vi "Ascensor_parcial1.vi"() -> ()   [LabVIEW 2018]
panel:
  in  "Enum":T1(ring)=enum."Cerrar"
  out "Asc/Desc":i16
  out "Pet Asc":i32[](array[numeric])
  out "Pet Desc":i32[](array[numeric])
  in  "Stop/Start":bool
  in  "Automatico/Manual":bool
  in  "stop":bool
  out "PurtasAux":dbl
  in  "Abierto M":bool
  in  "AbajoM":bool
  in  "Cerrado M":bool
  in  "Sen Puerta":bool
  in  "ArribaM":bool
  out "Elevador":i8(ring) caption="Puertas Elevador"
  in  "Down 2":bool
  in  "Up 2":bool
  in  "Down 3":bool
  in  "Up 3":bool
  in  "Down 4":bool
  in  "Up 1":bool
  in  "Close":bool
  in  "Open":bool
  in  "4":bool
  in  "1":bool
  in  "2":bool
  in  "3":bool
  in  "Display":i8(ring)
  out "Pos S3":i32=477
  out "Pos S4":i32=351
  out "Pos S2":i32=602
  out "Pos S1":i32=730
  in  "S4":bool
  in  "S3":bool
  in  "S2":bool
  in  "S1":bool
  # "Botonera interna"
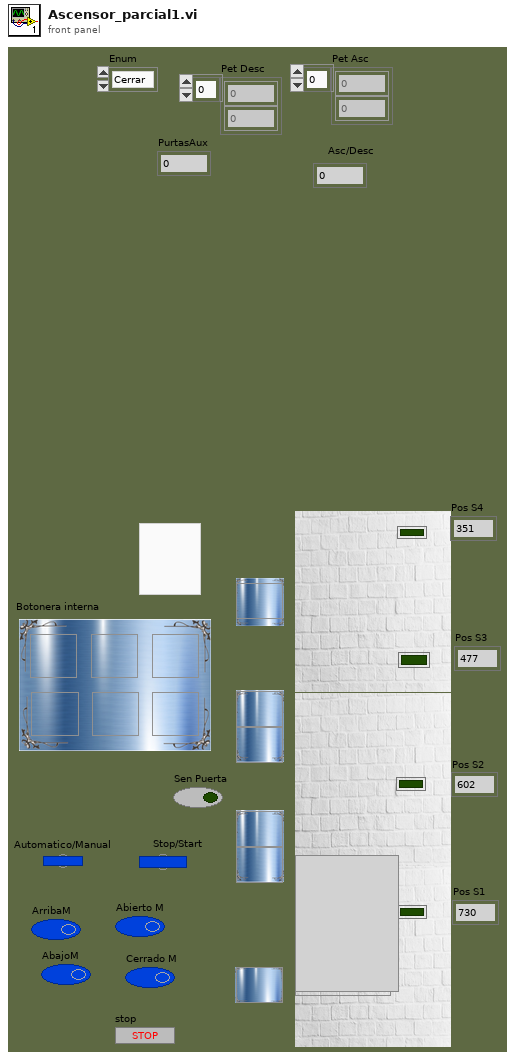
[diagram p1: front panel]
types:
  T1 = enum16{"Abrir", "Cerrar", "Ascender ", "Descender", "Eliminar"}
  T2 = enum16{"Abrir", "Cerrar", "Ascender ", "Descender", ""}
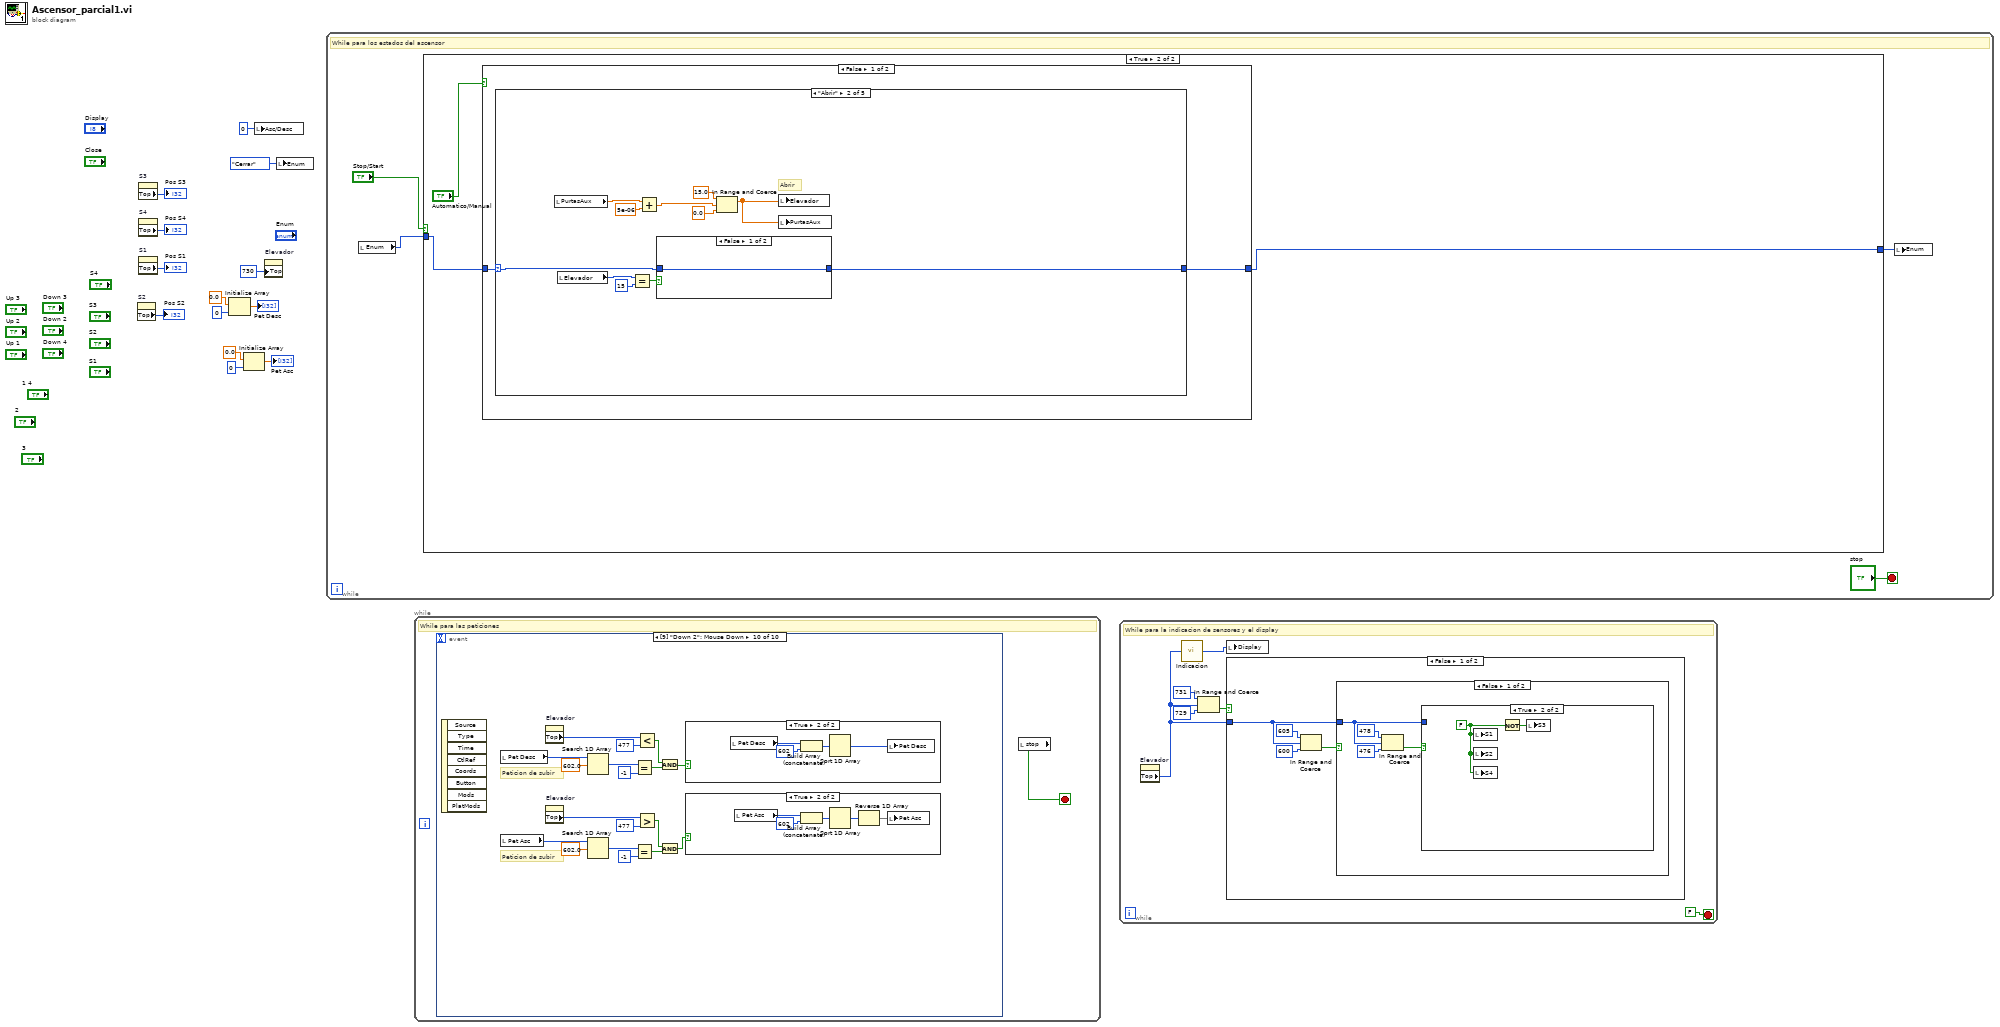
[diagram p0: block diagram]
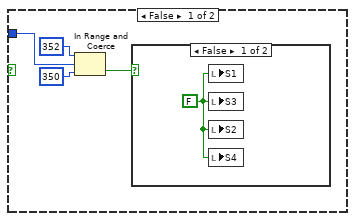
[diagram p2: hidden frame]
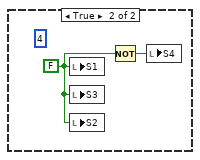
[diagram p3: hidden frame]
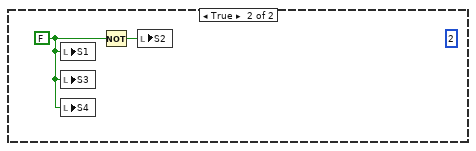
[diagram p4: hidden frame]
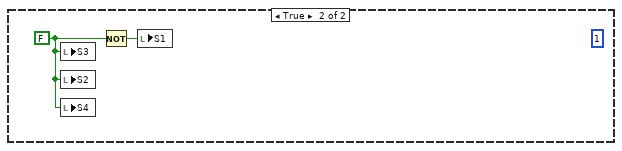
[diagram p5: hidden frame]
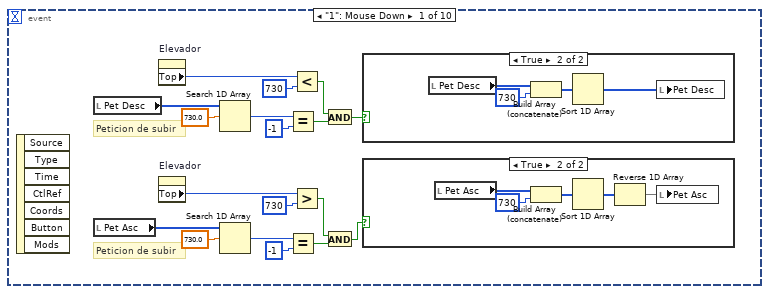
[diagram p6: hidden frame]
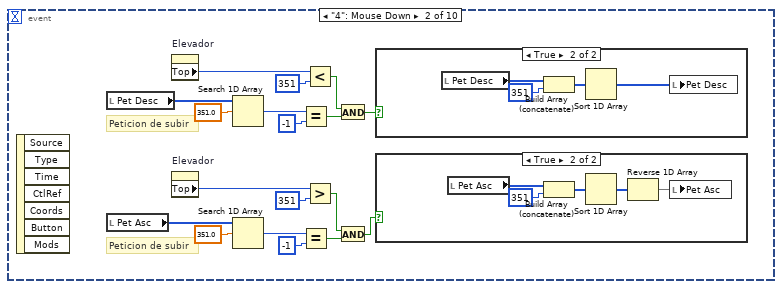
[diagram p9: hidden frame]
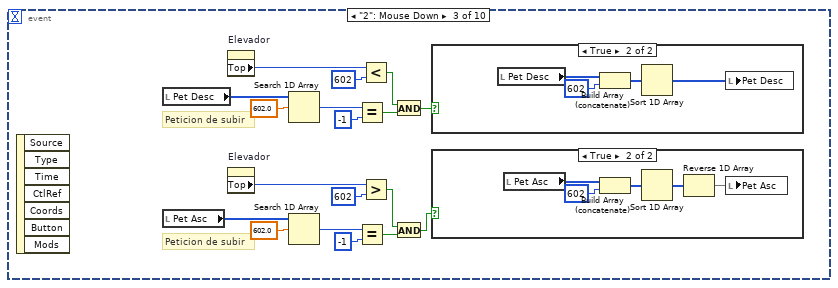
[diagram p12: hidden frame]
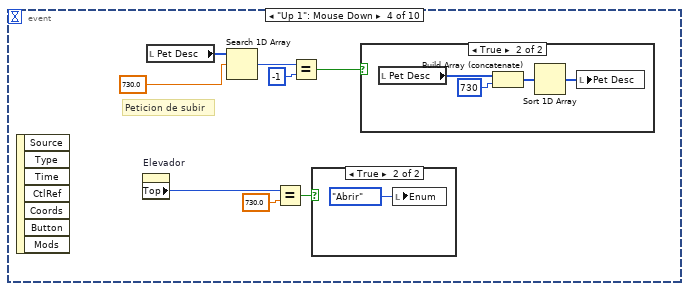
[diagram p15: hidden frame]
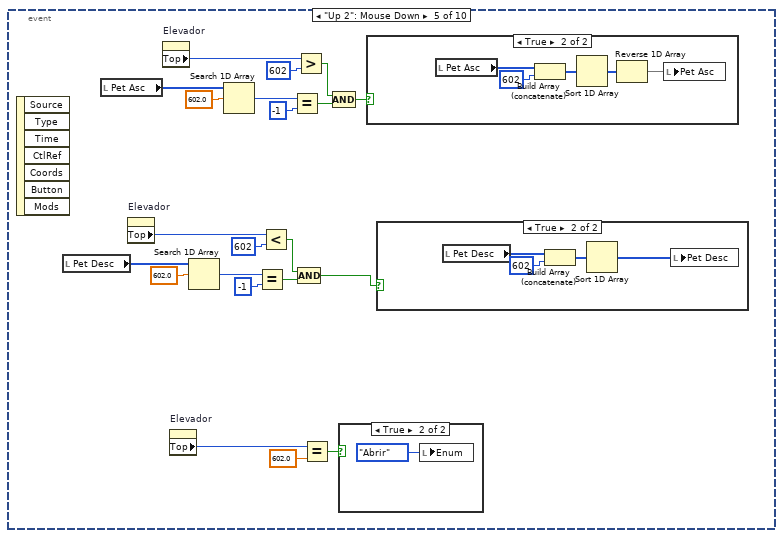
[diagram p18: hidden frame]
diagram:
  n1 = property on="S2" class="Bool (strict)"() -> ("Top"=→"Pos S2":i32)  [unwired: 2 in, 2 out]
  n2 = property on="S3" class="Bool (strict)"() -> ("Top"=→"Pos S3":i32)  [unwired: 2 in, 2 out]
  n3 = property on="S4" class="Bool (strict)"() -> ("Top"=→"Pos S4":i32)  [unwired: 2 in, 2 out]
  n4 = property on="S1" class="Bool (strict)"() -> ("Top"=→"Pos S1":i32)  [unwired: 2 in, 2 out]
  n5 = Initialize Array(0.0 ("element"), 0 ("dimension size")) -> (→"Pet Desc":dbl[])
  n6 = Initialize Array(0.0 ("element"), 0 ("dimension size")) -> (→"Pet Asc":dbl[])
  n7 = local write "Asc/Desc"(i16 0 ("Asc/Desc")) -> ()
  n8 = property on="Elevador" class="Ring (strict)"("Top"=730 ("Position:Top")) -> ()  [unwired: 2 in, 2 out]
  n9 = local write "Enum"(T1."Cerrar" ("Enum")) -> ()
  n10 = while {
    stop <- "stop" stop-if-true
    # "While para los estados del ascensor"
    n11 = local read "Enum"() -> (w15:T1)
    n12 = case shown="True" "Stop/Start" {
      tunnel: w15 -> [_ w20]
      tunnel: [T1."Cerrar" ("Enum") w19] -> w14
      frame False {
      }
      frame True {
        n13 = case shown="False" "Automatico/Manual" {
          tunnel: w20 -> [w22 _]
          tunnel: [w23 T1."Cerrar" ("Enum")] -> w19
          frame False {
            n14 = case shown="\"Abrir\"" w22 {
              selector: w22 -> [_ w42 w58 w73 w114]
              tunnel: [T1."Abrir" ("Enum") w43 w57 w72 w133] -> w23
              frame "Eliminar" {
                # "Eliminar"
                n15 = local read "Asc/Desc"() -> (w25:i16)
                n16 = case shown="1, Default" w25 {
                  frame 1, Default {
                    n17 = local read "Pet Asc"() -> (w33:i32[])
                    n18 = Delete From Array(array=w33, index=0) -> (array with subset deleted=w26:i32[])  [unwired: 1 in, 1 out]
                    n19 = local write "Pet Asc"(w26) -> ()
                    n20 = Array Size(array=w26) -> (size(s)=w31:i32)
                    n21 = Equal To 0?(x=w31) -> (x = 0?=w30:bool)
                    n22 = Select(t=0.0, s=w30, f=1.0 ("t")) -> (s? t:f=w29:dbl)
                    n23 = local write "Asc/Desc"(w29) -> ()
                  }
                  frame 2 {
                    n24 = local read "Pet Desc"() -> (w41:i32[])
                    n25 = Delete From Array(array=w41, index=0) -> (array with subset deleted=w39:i32[])  [unwired: 1 in, 1 out]
                    n26 = local write "Pet Desc"(w39) -> ()
                    n27 = Array Size(array=w39) -> (size(s)=w38:i32)
                    n28 = Equal To 0?(x=w38) -> (x = 0?=w37:bool)
                    n29 = Select(t=0.0, s=w37, f=2.0 ("t")) -> (s? t:f=w36:dbl)
                    n30 = local write "Asc/Desc"(w36) -> ()
                  }
                }
              }
              frame "Abrir" {
                # "Abrir"
                n31 = local read "PurtasAux"() -> (w51:dbl)
                n32 = local read "Elevador"() -> (w46:i8)
                n33 = Equal?(x=w46, y=i8 15) -> (x = y?=w44:bool)
                n34 = Add(x=w51, y=5e-06) -> (x+y=w52:dbl)
                n35 = case shown="False" w44 {
                  tunnel: [w53 T2."Cerrar"] -> w43
                  tunnel: w42 -> [w53 _]
                  frame False {
                  }
                  frame True {
                    n36 = Wait (ms)(milliseconds to wait=u32 1000) -> ()  [unwired: 1 out]
                  }
                }
                n37 = In Range and Coerce(upper limit=15.0, x=w52, lower limit=0.0 ("upper limit")) -> (coerced(x)=w47:dbl)  [unwired: 1 out]
                n38 = local write "Elevador"(w47) -> ()
                n39 = local write "PurtasAux"(w47) -> ()
              }
              frame "Descender" {
                # "Descender"
                n40 = local write "Asc/Desc"(i16 2 ("Asc/Desc")) -> ()
                n41 = local read "Pet Desc"() -> (w64:i32[])
                n42 = property on="Elevador" class="Ring (strict)"() -> ("Top"=w62:i32)  [unwired: 2 in, 2 out]
                n43 = property on="Elevador" class="Ring (strict)"() -> ("Top"=w67:i32)  [unwired: 2 in, 2 out]
                n44 = Index Array(array=w64) -> (element=w63:i32)  [unwired: 1 in]
                n45 = Equal?(x=w63, y=w62) -> (x = y?=w61:bool)
                n46 = Increment(x=w67) -> (x+1=w66:i32)
                n47 = case shown="False" w61 {
                  tunnel: [w68 T1."Eliminar" ("Enum")] -> w57
                  tunnel: w58 -> [w68 _]
                  frame False {
                  }
                  frame True {
                  }
                }
                n48 = In Range and Coerce(upper limit=730.0, x=w66, lower limit=351.0 ("upper limit")) -> (coerced(x)=w65:dbl)  [unwired: 1 out]
                n49 = property on="Elevador" class="Ring (strict)"("Top"=w65) -> ()  [unwired: 2 in, 2 out]
              }
              frame "Ascender " {
                # "Ascender"
                n50 = local read "Pet Asc"() -> (w77:i32[])
                n51 = property on="Elevador" class="Ring (strict)"() -> ("Top"=w81:i32)  [unwired: 2 in, 2 out]
                n52 = property on="Elevador" class="Ring (strict)"() -> ("Top"=w75:i32)  [unwired: 2 in, 2 out]
                n53 = Index Array(array=w77) -> (element=w76:i32)  [unwired: 1 in]
                n54 = Equal?(x=w76, y=w75) -> (x = y?=w74:bool)
                n55 = Decrement(x=w81) -> (x-1=w78:i32)
                n56 = case shown="False" w74 {
                  tunnel: [w82 T1."Eliminar" ("Enum")] -> w72
                  tunnel: w73 -> [w82 _]
                  frame False {
                  }
                  frame True {
                    n57 = property on="Elevador" class="Ring (strict)"() -> ("Top"=w84:i32)  [unwired: 2 in, 2 out]
                    n58 = Increment(x=w84) -> (x+1=w83:i32)
                    n59 = property on="Elevador" class="Ring (strict)"("Top"=w83) -> ()  [unwired: 2 in, 2 out]
                  }
                }
                n60 = In Range and Coerce(upper limit=730.0, x=w78, lower limit=351.0 ("upper limit")) -> (coerced(x)=w70:dbl)  [unwired: 1 out]
                n61 = property on="Elevador" class="Ring (strict)"("Top"=w70) -> ()  [unwired: 2 in, 2 out]
                "Asc/Desc" <- i16 1 ("Asc/Desc")
              }
              frame "Cerrar", Default {
                # "Cerrando"
                n62 = local read "PurtasAux"() -> (w110:dbl)
                n63 = local read "Pet Desc"() -> (w94:i32[])
                n64 = local read "Pet Desc"() -> (w120:i32[])
                n65 = local read "Pet Asc"() -> (w105:i32[])
                n66 = local read "Elevador"() -> (w117:i8)
                n67 = local read "Asc/Desc"() -> (w107:i16)
                n68 = local read "Asc/Desc"() -> (w91:i16)
                n69 = local read "Asc/Desc"() -> (w119:i16)
                n70 = Array Size(array=w105) -> (size(s)=w103:i32)
                n71 = Array Size(array=w94) -> (size(s)=w96:i32)
                n72 = Array Size(array=w120) -> (size(s)=w121:i32)
                n73 = Subtract(x=w110, y=5e-06) -> (x-y=w140:dbl)
                n74 = Not Equal To 0?(x=w103) -> (x != 0?=w104:bool)
                n75 = Not Equal To 0?(x=w96) -> (x != 0?=w95:bool)
                n76 = Not Equal To 0?(x=w121) -> (x != 0?=w124:bool)
                n77 = Equal?(x=w107, y=i8 0) -> (x = y?=w86:bool)
                n78 = Equal?(x=w91, y=i8 0) -> (x = y?=w93:bool)
                n79 = Equal?(x=w117, y=i8 0) -> (x = y?=w122:bool)
                n80 = Equal?(x=w119, y=i16 2) -> (x = y?=w123:bool)
                n81 = local read "Asc/Desc"() -> (w100:i16)
                n82 = local read "Asc/Desc"() -> (w99:i16)
                n83 = Compound Arithmetic op=AND(w122, w123, w124) -> (w115:bool)
                n84 = Compound Arithmetic op=AND(w86, w104) -> (w102:bool)
                n85 = Compound Arithmetic op=AND(w93, w95) -> (w97:bool)
                n86 = In Range and Coerce(upper limit=15.0, x=w140, lower limit=0.0 ("upper limit")) -> (coerced(x)=w111:dbl)  [unwired: 1 out]
                n87 = local read "Pet Asc"() -> (w129:i32[])
                n88 = case shown="False" w115 {
                  tunnel: w114 -> [w145 _]
                  tunnel: [w145 T2."Descender"] -> w113
                  frame False {
                  }
                  frame True {
                  }
                }
                n89 = Select(t=1.0, s=w102, f=w100) -> (s? t:f=w90:dbl)
                n90 = Select(t=2.0, s=w97, f=w99) -> (s? t:f=w89:dbl)
                n91 = local read "Elevador"() -> (w132:i8)
                n92 = local read "Asc/Desc"() -> (w130:i16)
                n93 = local write "PurtasAux"(w111) -> ()
                n94 = local write "Elevador"(w111) -> ()
                n95 = Add(x=w90, y=w89) -> (x+y=w88:dbl)
                n96 = Array Size(array=w129) -> (size(s)=w116:i32)
                n97 = To Long Integer(number=w88) -> (32bit integer=w87:i32)
                n98 = Not Equal To 0?(x=w116) -> (x != 0?=w126:bool)
                n99 = Equal?(x=w132, y=i8 0) -> (x = y?=w128:bool)
                n100 = Equal?(x=w130, y=i16 1) -> (x = y?=w127:bool)
                n101 = case shown="0, Default" w87 {
                  tunnel: w86 -> [_ w141 w143]
                  frame 0, Default {
                  }
                  frame 1 {
                    n102 = case shown="True" w141 {
                      frame False {
                      }
                      frame True {
                        n103 = local write "Asc/Desc"(i16 1 ("Asc/Desc")) -> ()
                      }
                    }
                  }
                  frame 2 {
                    n104 = case shown="False" w143 {
                      frame False {
                      }
                      frame True {
                        n105 = local write "Asc/Desc"(i16 2 ("Asc/Desc")) -> ()
                      }
                    }
                  }
                }
                n106 = Compound Arithmetic op=AND(w128, w127, w126) -> (w125:bool)
                n107 = case shown="False" w125 {
                  tunnel: w113 -> [w147 _]
                  tunnel: [w147 T2."Ascender "] -> w112
                  frame False {
                  }
                  frame True {
                  }
                }
                n108 = Or(x="Open", y="Sen Puerta") -> (x .or. y?=w136:bool)
                n109 = case shown="False" w136 {
                  tunnel: [w149 T2."Abrir"] -> w133
                  tunnel: w112 -> [w149 _]
                  frame False {
                  }
                  frame True {
                  }
                }
              }
            }
          }
          frame True {
            n110 = case shown="True" "Abierto M" {
              frame False {
                n111 = case shown="True" "Cerrado M" {
                  frame False {
                  }
                  frame True {
                    n112 = local read "PurtasAux"() -> (w155:dbl)
                    n113 = Subtract(x=w155, y=5e-06) -> (x-y=w160:dbl)
                    n114 = In Range and Coerce(upper limit=15.0, x=w160, lower limit=0.0 ("upper limit")) -> (coerced(x)=w156:dbl)  [unwired: 1 out]
                    "PurtasAux" <- w156
                    n115 = local write "Elevador"(w156) -> ()
                  }
                }
              }
              frame True {
                n116 = local read "PurtasAux"() -> (w162:dbl)
                n117 = Add(x=w162, y=5e-06) -> (x+y=w163:dbl)
                n118 = In Range and Coerce(upper limit=15.0, x=w163, lower limit=0.0 ("upper limit")) -> (coerced(x)=w161:dbl)  [unwired: 1 out]
                "Elevador" <- w161
                n119 = local write "PurtasAux"(w161) -> ()
              }
            }
            n120 = case shown="False" "ArribaM" {
              frame False {
                n121 = case shown="True" "AbajoM" {
                  frame False {
                  }
                  frame True {
                    n122 = property on="Elevador" class="Ring (strict)"() -> ("Top"=w172:i32)  [unwired: 2 in, 2 out]
                    n123 = Increment(x=w172) -> (x+1=w171:i32)
                    n124 = In Range and Coerce(upper limit=730.0, x=w171, lower limit=351.0 ("upper limit")) -> (coerced(x)=w170:dbl)  [unwired: 1 out]
                    n125 = property on="Elevador" class="Ring (strict)"("Top"=w170) -> ()  [unwired: 2 in, 2 out]
                  }
                }
              }
              frame True {
                n126 = property on="Elevador" class="Ring (strict)"() -> ("Top"=w177:i32)  [unwired: 2 in, 2 out]
                n127 = Decrement(x=w177) -> (x-1=w174:i32)
                n128 = In Range and Coerce(upper limit=730.0, x=w174, lower limit=351.0 ("upper limit")) -> (coerced(x)=w173:dbl)  [unwired: 1 out]
                n129 = property on="Elevador" class="Ring (strict)"("Top"=w173) -> ()  [unwired: 2 in, 2 out]
              }
            }
          }
        }
      }
    }
    n130 = local write "Enum"(w14) -> ()
  }
  n131 = while {
    stop <- w178 stop-if-true
    # "While para las peticiones"
    n132 = event shown="[9] \"Down 2\": Mouse Down" {
      selector: _ -> [_ _ _ _ _ _ _ _ _ _]
      dyn-events: _ -> [_ _ _ _ _ _ _ _ _ _]
      timeout: _ -> [_ _ _ _ _ _ _ _ _ _]
      event "1": Mouse Down {
        # "Peticion de subir"
        # "Peticion de subir"
        n133 = event-data() -> ()  [unwired: 1 in, 7 out]
        n134 = local read "Pet Desc"() -> (w193:i32[])
        n135 = local read "Pet Asc"() -> (w182:i32[])
        n136 = property on="Elevador" class="Ring (strict)"() -> ("Top"=w196:i32)  [unwired: 2 in, 2 out]
        n137 = property on="Elevador" class="Ring (strict)"() -> ("Top"=w179:i32)  [unwired: 2 in, 2 out]
        n138 = Search 1D Array(1D array=w193, element=730.0) -> (index of element=w192:i32)  [unwired: 1 in]
        n139 = Search 1D Array(1D array=w182, element=730.0) -> (index of element=w183:i32)  [unwired: 1 in]
        n140 = Equal?(x=w192, y=-1) -> (x = y?=w190:bool)
        n141 = Equal?(x=w183, y=-1) -> (x = y?=w185:bool)
        n142 = Less?(x=w196, y=730) -> (x < y?=w189:bool)
        n143 = Greater?(x=w179, y=730) -> (0:w186:bool)
        n144 = And(x=w189, y=w190) -> (x .and. y?=w188:bool)
        n145 = And(x=w186, y=w185) -> (x .and. y?=w187:bool)
        n146 = case shown="True" w188 {
          frame False {
          }
          frame True {
            n147 = local read "Pet Desc"() -> (w205:i32[])
            n148 = Build Array (concatenate)(w205, 730 ("y")) -> (w203:i32[])
            n149 = Sort 1D Array(array=w203) -> (sorted array=w202:i32[])
            n150 = local write "Pet Desc"(w202) -> ()
          }
        }
        n151 = case shown="True" w187 {
          frame False {
          }
          frame True {
            n152 = local read "Pet Asc"() -> (w201:i32[])
            n153 = Build Array (concatenate)(w201, 730 ("y")) -> (w199:i32[])
            n154 = Sort 1D Array(array=w199) -> (sorted array=w198:i32[])
            n155 = Reverse 1D Array(array=w198) -> (reversed array=w197:i32[])
            n156 = local write "Pet Asc"(w197) -> ()
          }
        }
      }
      event "4": Mouse Down {
        # "Peticion de subir"
        # "Peticion de subir"
        n157 = event-data() -> ()  [unwired: 1 in, 7 out]
        n158 = local read "Pet Desc"() -> (w220:i32[])
        n159 = local read "Pet Asc"() -> (w209:i32[])
        n160 = property on="Elevador" class="Ring (strict)"() -> ("Top"=w223:i32)  [unwired: 2 in, 2 out]
        n161 = property on="Elevador" class="Ring (strict)"() -> ("Top"=w206:i32)  [unwired: 2 in, 2 out]
        n162 = Search 1D Array(1D array=w220, element=351.0) -> (index of element=w219:i32)  [unwired: 1 in]
        n163 = Search 1D Array(1D array=w209, element=351.0) -> (index of element=w210:i32)  [unwired: 1 in]
        n164 = Equal?(x=w219, y=-1) -> (x = y?=w217:bool)
        n165 = Equal?(x=w210, y=-1) -> (x = y?=w212:bool)
        n166 = Less?(x=w223, y=351) -> (x < y?=w216:bool)
        n167 = Greater?(x=w206, y=351) -> (0:w213:bool)
        n168 = And(x=w216, y=w217) -> (x .and. y?=w215:bool)
        n169 = And(x=w213, y=w212) -> (x .and. y?=w214:bool)
        n170 = case shown="True" w215 {
          frame False {
          }
          frame True {
            n171 = local read "Pet Desc"() -> (w232:i32[])
            n172 = Build Array (concatenate)(w232, 351 ("y")) -> (w230:i32[])
            n173 = Sort 1D Array(array=w230) -> (sorted array=w229:i32[])
            n174 = local write "Pet Desc"(w229) -> ()
          }
        }
        n175 = case shown="True" w214 {
          frame False {
          }
          frame True {
            n176 = local read "Pet Asc"() -> (w228:i32[])
            n177 = Build Array (concatenate)(w228, 351 ("y")) -> (w226:i32[])
            n178 = Sort 1D Array(array=w226) -> (sorted array=w225:i32[])
            n179 = Reverse 1D Array(array=w225) -> (reversed array=w224:i32[])
            n180 = local write "Pet Asc"(w224) -> ()
          }
        }
      }
      event "2": Mouse Down {
        # "Peticion de subir"
        # "Peticion de subir"
        n181 = event-data() -> ()  [unwired: 1 in, 7 out]
        n182 = local read "Pet Desc"() -> (w247:i32[])
        n183 = local read "Pet Asc"() -> (w236:i32[])
        n184 = property on="Elevador" class="Ring (strict)"() -> ("Top"=w250:i32)  [unwired: 2 in, 2 out]
        n185 = property on="Elevador" class="Ring (strict)"() -> ("Top"=w233:i32)  [unwired: 2 in, 2 out]
        n186 = Search 1D Array(1D array=w247, element=602.0) -> (index of element=w246:i32)  [unwired: 1 in]
        n187 = Search 1D Array(1D array=w236, element=602.0) -> (index of element=w237:i32)  [unwired: 1 in]
        n188 = Equal?(x=w246, y=-1) -> (x = y?=w244:bool)
        n189 = Equal?(x=w237, y=-1) -> (x = y?=w239:bool)
        n190 = Less?(x=w250, y=602) -> (x < y?=w243:bool)
        n191 = Greater?(x=w233, y=602) -> (0:w240:bool)
        n192 = And(x=w243, y=w244) -> (x .and. y?=w242:bool)
        n193 = And(x=w240, y=w239) -> (x .and. y?=w241:bool)
        n194 = case shown="True" w242 {
          frame False {
          }
          frame True {
            n195 = local read "Pet Desc"() -> (w256:i32[])
            n196 = Build Array (concatenate)(w256, 602 ("y")) -> (w258:i32[])
            n197 = Sort 1D Array(array=w258) -> (sorted array=w257:i32[])
            n198 = local write "Pet Desc"(w257) -> ()
          }
        }
        n199 = case shown="True" w241 {
          frame False {
          }
          frame True {
            n200 = local read "Pet Asc"() -> (w255:i32[])
            n201 = Build Array (concatenate)(w255, 602 ("y")) -> (w253:i32[])
            n202 = Sort 1D Array(array=w253) -> (sorted array=w252:i32[])
            n203 = Reverse 1D Array(array=w252) -> (reversed array=w251:i32[])
            n204 = local write "Pet Asc"(w251) -> ()
          }
        }
      }
      event "Up 1": Mouse Down {
        # "Peticion de subir"
        n205 = event-data() -> ()  [unwired: 1 in, 7 out]
        n206 = property on="Elevador" class="Ring (strict)"() -> ("Top"=w261:i32)  [unwired: 2 in, 2 out]
        n207 = local read "Pet Desc"() -> (w266:i32[])
        n208 = Search 1D Array(1D array=w266, element=730.0) -> (index of element=w265:i32)  [unwired: 1 in]
        n209 = Equal?(x=w261, y=730.0 ("element")) -> (x = y?=w260:bool)
        n210 = Equal?(x=w265, y=-1) -> (x = y?=w263:bool)
        n211 = case shown="True" w260 {
          frame False {
          }
          frame True {
            n212 = local write "Enum"(T1."Abrir" ("Enum")) -> ()
          }
        }
        n213 = case shown="True" w263 {
          frame False {
          }
          frame True {
            n214 = local read "Pet Desc"() -> (w272:i32[])
            n215 = Build Array (concatenate)(w272, 730 ("y")) -> (w270:i32[])
            n216 = Sort 1D Array(array=w270) -> (sorted array=w269:i32[])
            n217 = local write "Pet Desc"(w269) -> ()
          }
        }
      }
      event "Up 2": Mouse Down {
        n218 = event-data() -> ()  [unwired: 1 in, 7 out]
        n219 = local read "Pet Desc"() -> (w280:i32[])
        n220 = local read "Pet Asc"() -> (w290:i32[])
        n221 = property on="Elevador" class="Ring (strict)"() -> ("Top"=w277:i32)  [unwired: 2 in, 2 out]
        n222 = property on="Elevador" class="Ring (strict)"() -> ("Top"=w293:i32)  [unwired: 2 in, 2 out]
        n223 = property on="Elevador" class="Ring (strict)"() -> ("Top"=w275:i32)  [unwired: 2 in, 2 out]
        n224 = Search 1D Array(1D array=w280, element=602.0) -> (index of element=w281:i32)  [unwired: 1 in]
        n225 = Search 1D Array(1D array=w290, element=602.0) -> (index of element=w289:i32)  [unwired: 1 in]
        n226 = Equal?(x=w281, y=-1) -> (x = y?=w283:bool)
        n227 = Less?(x=w277, y=602) -> (x < y?=w284:bool)
        n228 = Equal?(x=w289, y=-1) -> (x = y?=w287:bool)
        n229 = Greater?(x=w293, y=602) -> (0:w286:bool)
        n230 = Compound Arithmetic op=AND(w284, w283) -> (w276:bool)
        n231 = Equal?(x=w275, y=602.0 ("element")) -> (x = y?=w274:bool)
        n232 = Compound Arithmetic op=AND(w286, w287) -> (w285:bool)
        n233 = case shown="True" w274 {
          frame False {
          }
          frame True {
            n234 = local write "Enum"(T1."Abrir" ("Enum")) -> ()
          }
        }
        n235 = case shown="True" w285 {
          frame False {
          }
          frame True {
            n236 = local read "Pet Asc"() -> (w303:i32[])
            n237 = Build Array (concatenate)(w303, 602 ("y")) -> (w301:i32[])
            n238 = Sort 1D Array(array=w301) -> (sorted array=w299:i32[])
            n239 = Reverse 1D Array(array=w299) -> (reversed array=w300:i32[])
            n240 = local write "Pet Asc"(w300) -> ()
          }
        }
        n241 = case shown="True" w276 {
          frame False {
          }
          frame True {
            n242 = local read "Pet Desc"() -> (w298:i32[])
            n243 = Build Array (concatenate)(w298, 602 ("y")) -> (w296:i32[])
            n244 = Sort 1D Array(array=w296) -> (sorted array=w295:i32[])
            n245 = local write "Pet Desc"(w295) -> ()
          }
        }
      }
      event "Up 3": Mouse Down {
        n246 = event-data() -> ()  [unwired: 1 in, 8 out]
        n247 = local read "Pet Desc"() -> (w315:i32[])
        n248 = local read "Pet Asc"() -> (w323:i32[])
        n249 = property on="Elevador" class="Ring (strict)"() -> ("Top"=w314:i32)  [unwired: 2 in, 2 out]
        n250 = property on="Elevador" class="Ring (strict)"() -> ("Top"=w324:i32)  [unwired: 2 in, 2 out]
        n251 = property on="Elevador" class="Ring (strict)"() -> ("Top"=w312:i32)  [unwired: 2 in, 2 out]
        n252 = Search 1D Array(1D array=w315, element=477.0) -> (index of element=w316:i32)  [unwired: 1 in]
        n253 = Search 1D Array(1D array=w323, element=477.0) -> (index of element=w322:i32)  [unwired: 1 in]
        n254 = Equal?(x=w316, y=-1) -> (x = y?=w317:bool)
        n255 = Less?(x=w314, y=477) -> (x < y?=w318:bool)
        n256 = Equal?(x=w322, y=-1) -> (x = y?=w321:bool)
        n257 = Greater?(x=w324, y=477) -> (0:w320:bool)
        n258 = Compound Arithmetic op=AND(w318, w317) -> (w313:bool)
        n259 = Equal?(x=w312, y=477.0 ("element")) -> (x = y?=w304:bool)
        n260 = Compound Arithmetic op=AND(w320, w321) -> (w319:bool)
        n261 = case shown="False" w304 {
          frame False {
          }
          frame True {
            n262 = local write "Enum"(T1."Abrir" ("Enum")) -> ()
          }
        }
        n263 = case shown="True" w319 {
          frame False {
          }
          frame True {
            n264 = local read "Pet Asc"() -> (w334:i32[])
            n265 = Build Array (concatenate)(w334, 477 ("y")) -> (w332:i32[])
            n266 = Sort 1D Array(array=w332) -> (sorted array=w331:i32[])
            n267 = Reverse 1D Array(array=w331) -> (reversed array=w330:i32[])
            n268 = local write "Pet Asc"(w330) -> ()
          }
        }
        n269 = case shown="True" w313 {
          frame False {
          }
          frame True {
            n270 = local read "Pet Desc"() -> (w329:i32[])
            n271 = Build Array (concatenate)(w329, 477 ("y")) -> (w327:i32[])
            n272 = Sort 1D Array(array=w327) -> (sorted array=w326:i32[])
            n273 = local write "Pet Desc"(w326) -> ()
          }
        }
      }
      event "Down 4": Mouse Down {
        # "Peticion de subir"
        n274 = event-data() -> ()  [unwired: 1 in, 8 out]
        n275 = property on="Elevador" class="Ring (strict)"() -> ("Top"=w339:i32)  [unwired: 2 in, 2 out]
        n276 = local read "Pet Asc"() -> (w342:i32[])
        n277 = Search 1D Array(1D array=w342, element=351.0) -> (index of element=w341:i32)  [unwired: 1 in]
        n278 = Equal?(x=w339, y=351.0 ("element")) -> (x = y?=w338:bool)
        n279 = Equal?(x=w341, y=-1) -> (x = y?=w340:bool)
        n280 = case shown="True" w338 {
          frame False {
          }
          frame True {
            n281 = local write "Enum"(T1."Abrir" ("Enum")) -> ()
          }
        }
        n282 = case shown="True" w340 {
          frame False {
          }
          frame True {
            n283 = local read "Pet Asc"() -> (w348:i32[])
            n284 = Build Array (concatenate)(w348, 351 ("y")) -> (w346:i32[])
            n285 = Sort 1D Array(array=w346) -> (sorted array=w345:i32[])
            n286 = Reverse 1D Array(array=w345) -> (reversed array=w344:i32[])
            n287 = local write "Pet Asc"(w344) -> ()
          }
        }
      }
      event "3": Mouse Down {
        # "Peticion de subir"
        # "Peticion de subir"
        n288 = event-data() -> ()  [unwired: 1 in, 7 out]
        n289 = local read "Pet Desc"() -> (w363:i32[])
        n290 = local read "Pet Asc"() -> (w352:i32[])
        n291 = property on="Elevador" class="Ring (strict)"() -> ("Top"=w366:i32)  [unwired: 2 in, 2 out]
        n292 = property on="Elevador" class="Ring (strict)"() -> ("Top"=w349:i32)  [unwired: 2 in, 2 out]
        n293 = Search 1D Array(1D array=w363, element=477.0) -> (index of element=w362:i32)  [unwired: 1 in]
        n294 = Search 1D Array(1D array=w352, element=477.0) -> (index of element=w353:i32)  [unwired: 1 in]
        n295 = Equal?(x=w362, y=-1) -> (x = y?=w360:bool)
        n296 = Equal?(x=w353, y=-1) -> (x = y?=w355:bool)
        n297 = Less?(x=w366, y=477) -> (x < y?=w359:bool)
        n298 = Greater?(x=w349, y=477) -> (0:w356:bool)
        n299 = And(x=w359, y=w360) -> (x .and. y?=w358:bool)
        n300 = And(x=w356, y=w355) -> (x .and. y?=w357:bool)
        n301 = case shown="True" w358 {
          frame False {
          }
          frame True {
            n302 = local read "Pet Desc"() -> (w375:i32[])
            n303 = Build Array (concatenate)(w375, 477 ("y")) -> (w373:i32[])
            n304 = Sort 1D Array(array=w373) -> (sorted array=w372:i32[])
            n305 = local write "Pet Desc"(w372) -> ()
          }
        }
        n306 = case shown="True" w357 {
          frame False {
          }
          frame True {
            n307 = local read "Pet Asc"() -> (w371:i32[])
            n308 = Build Array (concatenate)(w371, 477 ("y")) -> (w369:i32[])
            n309 = Sort 1D Array(array=w369) -> (sorted array=w368:i32[])
            n310 = Reverse 1D Array(array=w368) -> (reversed array=w367:i32[])
            n311 = local write "Pet Asc"(w367) -> ()
          }
        }
      }
      event "Down 3": Mouse Down {
        n312 = event-data() -> ()  [unwired: 1 in, 8 out]
        n313 = local read "Pet Asc"() -> (w387:i32[])
        n314 = local read "Pet Desc"() -> (w395:i32[])
        n315 = property on="Elevador" class="Ring (strict)"() -> ("Top"=w386:i32)  [unwired: 2 in, 2 out]
        n316 = property on="Elevador" class="Ring (strict)"() -> ("Top"=w396:i32)  [unwired: 2 in, 2 out]
        n317 = property on="Elevador" class="Ring (strict)"() -> ("Top"=w384:i32)  [unwired: 2 in, 2 out]
        n318 = Search 1D Array(1D array=w387, element=477.0) -> (index of element=w388:i32)  [unwired: 1 in]
        n319 = Search 1D Array(1D array=w395, element=477.0) -> (index of element=w394:i32)  [unwired: 1 in]
        n320 = Equal?(x=w388, y=-1) -> (x = y?=w389:bool)
        n321 = Greater?(x=w386, y=477) -> (0:w390:bool)
        n322 = Equal?(x=w394, y=-1) -> (x = y?=w393:bool)
        n323 = Less?(x=w396, y=477) -> (x < y?=w392:bool)
        n324 = Compound Arithmetic op=AND(w390, w389) -> (w385:bool)
        n325 = Equal?(x=w384, y=477.0 ("element")) -> (x = y?=w383:bool)
        n326 = Compound Arithmetic op=AND(w392, w393) -> (w391:bool)
        n327 = case shown="True" w383 {
          frame False {
          }
          frame True {
            n328 = local write "Enum"(T1."Abrir" ("Enum")) -> ()
          }
        }
        n329 = case shown="True" w391 {
          frame False {
          }
          frame True {
            n330 = local read "Pet Desc"() -> (w406:i32[])
            n331 = Build Array (concatenate)(w406, 477 ("y")) -> (w404:i32[])
            n332 = Sort 1D Array(array=w404) -> (sorted array=w403:i32[])
            n333 = local write "Pet Desc"(w403) -> ()
          }
        }
        n334 = case shown="True" w385 {
          frame False {
          }
          frame True {
            n335 = local read "Pet Asc"() -> (w402:i32[])
            n336 = Build Array (concatenate)(w402, 477 ("y")) -> (w400:i32[])
            n337 = Sort 1D Array(array=w400) -> (sorted array=w399:i32[])
            n338 = Reverse 1D Array(array=w399) -> (reversed array=w398:i32[])
            n339 = local write "Pet Asc"(w398) -> ()
          }
        }
      }
      event "Down 2": Mouse Down {
        # "Peticion de subir"
        # "Peticion de subir"
        n340 = event-data() -> ()  [unwired: 1 in, 8 out]
        n341 = local read "Pet Desc"() -> (w423:i32[])
        n342 = local read "Pet Asc"() -> (w414:i32[])
        n343 = property on="Elevador" class="Ring (strict)"() -> ("Top"=w424:i32)  [unwired: 2 in, 2 out]
        n344 = property on="Elevador" class="Ring (strict)"() -> ("Top"=w413:i32)  [unwired: 2 in, 2 out]
        n345 = Search 1D Array(1D array=w423, element=602.0) -> (index of element=w422:i32)  [unwired: 1 in]
        n346 = Search 1D Array(1D array=w414, element=602.0) -> (index of element=w415:i32)  [unwired: 1 in]
        n347 = Equal?(x=w422, y=-1) -> (x = y?=w421:bool)
        n348 = Equal?(x=w415, y=-1) -> (x = y?=w416:bool)
        n349 = Less?(x=w424, y=477) -> (x < y?=w420:bool)
        n350 = Greater?(x=w413, y=477) -> (0:w417:bool)
        n351 = And(x=w420, y=w421) -> (x .and. y?=w419:bool)
        n352 = And(x=w417, y=w416) -> (x .and. y?=w418:bool)
        n353 = case shown="True" w419 {
          frame False {
          }
          frame True {
            n354 = local read "Pet Desc"() -> (w433:i32[])
            n355 = Build Array (concatenate)(w433, 602 ("y")) -> (w431:i32[])
            n356 = Sort 1D Array(array=w431) -> (sorted array=w430:i32[])
            n357 = local write "Pet Desc"(w430) -> ()
          }
        }
        n358 = case shown="True" w418 {
          frame False {
          }
          frame True {
            n359 = local read "Pet Asc"() -> (w429:i32[])
            n360 = Build Array (concatenate)(w429, 602 ("y")) -> (w427:i32[])
            n361 = Sort 1D Array(array=w427) -> (sorted array=w426:i32[])
            n362 = Reverse 1D Array(array=w426) -> (reversed array=w425:i32[])
            n363 = local write "Pet Asc"(w425) -> ()
          }
        }
      }
    }
    n364 = local read "stop"() -> (w178:bool)
  }
  n365 = while {
    stop <- FALSE stop-if-true
    # "While para la indicacion de sensores y el display"
    n366 = property on="Elevador" class="Ring (strict)"() -> ("Top"=w434:i32)  [unwired: 2 in, 2 out]
    n367 = call "Indicacion.vi"("Pos Elevator"=w434) -> ("Indicacion"=w438:i32)
    n368 = In Range and Coerce(upper limit=731, x=w434, lower limit=729 ("upper limit")) -> (In Range?=w437:bool)  [unwired: 1 out]
    n369 = local write "Display"(w438) -> ()
    n370 = case shown="False" w437 {
      tunnel: w434 -> [w440 _]
      frame False {
        n371 = In Range and Coerce(upper limit=605, x=w440, lower limit=600 ("upper limit")) -> (In Range?=w441:bool)  [unwired: 1 out]
        n372 = case shown="False" w441 {
          tunnel: w440 -> [w444 _]
          frame False {
            n373 = In Range and Coerce(upper limit=478, x=w444, lower limit=476 ("upper limit")) -> (In Range?=w445:bool)  [unwired: 1 out]
            n374 = case shown="True" w445 {
              tunnel: w444 -> [w448 _]
              frame False {
                n375 = In Range and Coerce(upper limit=352, x=w448, lower limit=350 ("upper limit")) -> (In Range?=w449:bool)  [unwired: 1 out]
                n376 = case shown="False" w449 {
                  frame False {
                    w452 = FALSE ("S4")
                    n377 = local write "S1"(w452) -> ()
                    n378 = local write "S3"(w452) -> ()
                    n379 = local write "S2"(w452) -> ()
                    n380 = local write "S4"(w452) -> ()
                  }
                  frame True {
                    w453 = FALSE ("S4")
                    (unwired) 4 ("upper limit")
                    n381 = local write "S1"(w453) -> ()
                    n382 = local write "S3"(w453) -> ()
                    n383 = local write "S2"(w453) -> ()
                    n384 = Not(x=w453) -> (.not. x?=w454:bool)
                    n385 = local write "S4"(w454) -> ()
                  }
                }
              }
              frame True {
                w455 = FALSE ("S4")
                n386 = local write "S1"(w455) -> ()
                n387 = local write "S2"(w455) -> ()
                n388 = local write "S4"(w455) -> ()
                n389 = Not(x=w455) -> (.not. x?=w456:bool)
                n390 = local write "S3"(w456) -> ()
              }
            }
          }
          frame True {
            w458 = FALSE ("S4")
            (unwired) 2 ("upper limit")
            n391 = local write "S1"(w458) -> ()
            n392 = local write "S3"(w458) -> ()
            n393 = local write "S4"(w458) -> ()
            n394 = Not(x=w458) -> (.not. x?=w457:bool)
            n395 = local write "S2"(w457) -> ()
          }
        }
      }
      frame True {
        w460 = FALSE ("S4")
        (unwired) 1 ("upper limit")
        n396 = local write "S3"(w460) -> ()
        n397 = local write "S2"(w460) -> ()
        n398 = local write "S4"(w460) -> ()
        n399 = Not(x=w460) -> (.not. x?=w459:bool)
        n400 = local write "S1"(w459) -> ()
      }
    }
  }
